vi "LUT.hot-cold.vi"() -> (0 "Palette":cluster{u8, u8, u8}[](array[cluster]))   [LabVIEW 2013]
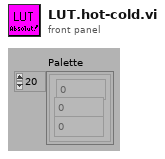
[diagram p1: front panel]
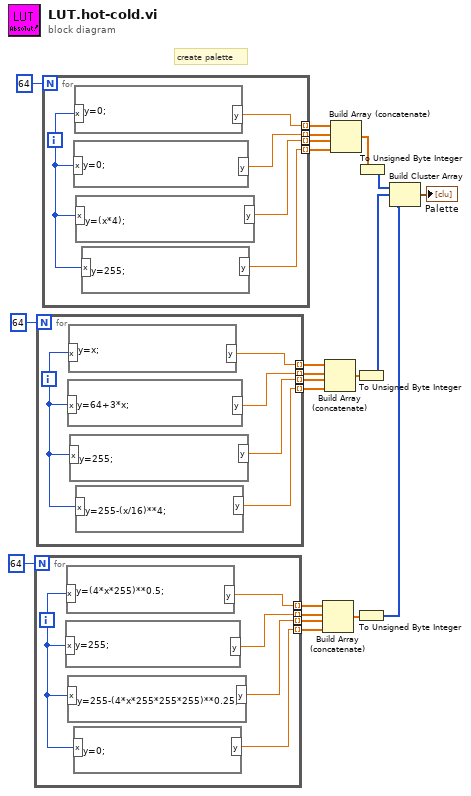
[diagram p0: block diagram]
diagram:
  # "create palette"
  n1 = for {
    N: 64 -> [_]
    tunnel: [w27] -> w7 mode=indexing
    tunnel: [w26] -> w6 mode=indexing
    tunnel: [w25] -> w5 mode=indexing
    tunnel: [w24] -> w4 mode=indexing
    i -> [w23]
    n2 = formula code="y=255;"("x"=w23) -> ("y"=w26:dbl)
    n3 = formula code="y=(4*x*255)**0.5;"("x"=w23) -> ("y"=w27:dbl)
    n4 = formula code="y=255-(4*x*255*255*255)**0.25;"("x"=w23) -> ("y"=w25:dbl)
    n5 = formula code="y=0;"("x"=w23) -> ("y"=w24:dbl)
  }
  n6 = for {
    N: 64 -> [_]
    tunnel: [w32] -> w14 mode=indexing
    tunnel: [w31] -> w13 mode=indexing
    tunnel: [w30] -> w12 mode=indexing
    tunnel: [w29] -> w11 mode=indexing
    i -> [w28]
    n7 = formula code="y=64+3*x;"("x"=w28) -> ("y"=w31:dbl)
    n8 = formula code="y=x;"("x"=w28) -> ("y"=w32:dbl)
    n9 = formula code="y=255;"("x"=w28) -> ("y"=w30:dbl)
    n10 = formula code="y=255-(x/16)**4;"("x"=w28) -> ("y"=w29:dbl)
  }
  n11 = for {
    N: 64 -> [_]
    tunnel: [w37] -> w21 mode=indexing
    tunnel: [w36] -> w20 mode=indexing
    tunnel: [w35] -> w19 mode=indexing
    tunnel: [w34] -> w18 mode=indexing
    i -> [w33]
    n12 = formula code="y=0;"("x"=w33) -> ("y"=w36:dbl)
    n13 = formula code="y=0;"("x"=w33) -> ("y"=w37:dbl)
    n14 = formula code="y=(x*4);"("x"=w33) -> ("y"=w35:dbl)
    n15 = formula code="y=255;"("x"=w33) -> ("y"=w34:dbl)
  }
  n16 = Build Array (concatenate)(w7, w6, w5, w4) -> (w3:dbl[])
  n17 = Build Array (concatenate)(w14, w13, w12, w11) -> (w10:dbl[])
  n18 = Build Array (concatenate)(w21, w20, w19, w18) -> (w17:dbl[])
  n19 = To Unsigned Byte Integer(number=w10) -> (unsigned 8bit integer=w9:u8[])
  n20 = To Unsigned Byte Integer(number=w3) -> (unsigned 8bit integer=w2:u8[])
  n21 = To Unsigned Byte Integer(number=w17) -> (unsigned 8bit integer=w16:u8[])
  n22 = Build Cluster Array(w16, w9, w2) -> (→"Palette":cluster{"y":u8, "y":u8, "y":u8}[])
